vi "Remove NaN from Array.vi"(1 "Input array":dbl[](array[numeric])) -> (0 "Array with values deleted":dbl[](array[numeric]))   [LabVIEW 2018, in "ASI TG-1000.lvlib"]
uses:
  ASI TG-1000.lvlib
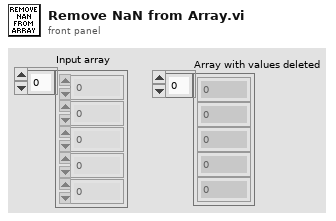
[diagram p1: front panel]
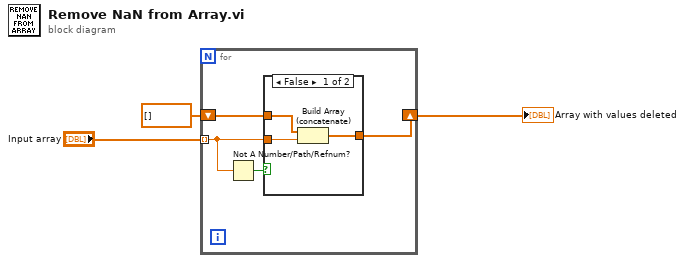
[diagram p0: block diagram]
diagram:
  n1 = for {
    tunnel: "Input array" -> [w4] mode=indexing
    shift-right: [w7] -> w1
    shift-left: dbl[] [] -> [w6]
    n2 = Not A Number/Path/Refnum?(number/path/refnum=w4) -> (NaN/Path/Refnum?=w5:bool)
    n3 = case shown="False" w5 {
      tunnel: w4 -> [w10 _]
      tunnel: [w9 w11] -> w7
      tunnel: w6 -> [w8 w11]
      frame False {
        n4 = Build Array (concatenate)(w8, w10) -> (w9:dbl[])
      }
      frame True {
      }
    }
  }
  "Array with values deleted" <- w1
